vi "solar_log EnQ.vi"(8 "error in (no error)":errorcluster, 9 "Front? (F)":bool, 10 "MSG":string, 11 "Create? (F)":bool) -> (0 "error out":errorcluster, 2 "Created New?":bool, 3 "LogQ":refnum<queue>)   [LabVIEW 2018]
doc: "This obtains and enqueues a message to the logger process. This VI is non-reentrant to avoid multiple opening multiple queue references."
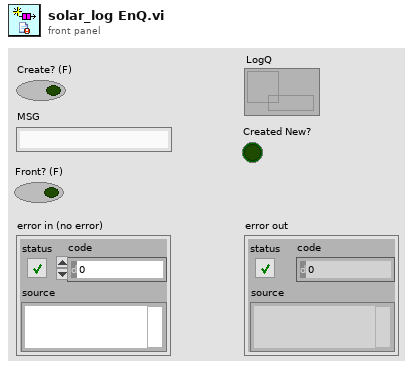
[diagram p1: front panel]
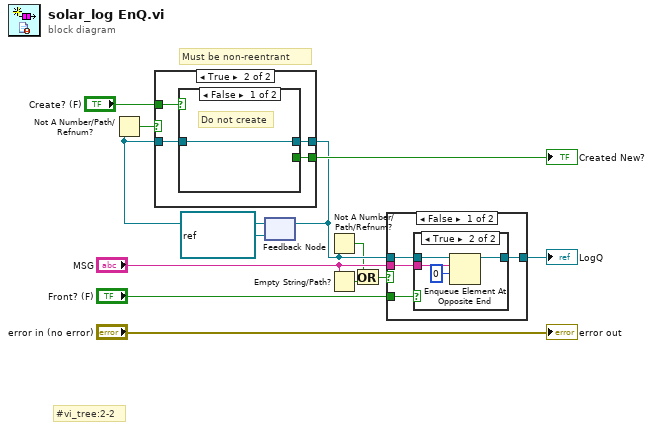
[diagram p0: block diagram]
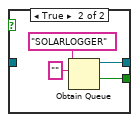
[diagram p3: hidden frame]
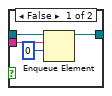
[diagram p4: hidden frame]
diagram:
  # "#vi_tree:2-2"
  # "Must be non-reentrant"
  n1 = feedback #1(refnum<queue> refnum ("queue out")) -> (w12:refnum<queue>)
  n2 = Not A Number/Path/Refnum?(number/path/refnum=w12) -> (NaN/Path/Refnum?=w3:bool)
  n3 = case shown="True" w3 {
    tunnel: [_ w18] -> w13
    tunnel: [w14 w17] -> w9
    tunnel: w12 -> [w14 w15]
    tunnel: "Create? (F)" -> [_ w16]
    frame False {
    }
    frame True {
      n4 = case shown="False" w16 {
        tunnel: [_ w21] -> w18
        tunnel: [w19 w20] -> w17
        tunnel: w15 -> [w19 _]
        frame False {
          # "Do not create"
        }
        frame True {
          n5 = Obtain Queue(name (unnamed)="SOLARLOGGER", element data type="") -> (queue out=w20:refnum<queue>, created new?=w21:bool)  [unwired: 3 in, 1 out]
        }
      }
    }
  }
  "Created New?" <- w13
  n6 = feedback-in #1(w9) -> ()
  n7 = Not A Number/Path/Refnum?(number/path/refnum=w9) -> (NaN/Path/Refnum?=w6:bool)
  n8 = Empty String/Path?(string/path="MSG") -> (empty?=w7:bool)
  n9 = Or(x=w6, y=w7) -> (x .or. y?=w5:bool)
  n10 = case shown="False" w5 {
    tunnel: "MSG" -> [w27 _]
    tunnel: [w26 w36] -> w1
    tunnel: w9 -> [w25 w36]
    tunnel: "Front? (F)" -> [w24 _]
    frame False {
      n11 = case shown="True" w24 {
        tunnel: w27 -> [w30 w33]
        tunnel: [w29 w34] -> w26
        tunnel: w25 -> [w28 w35]
        frame False {
          n12 = Enqueue Element(queue=w28, element=w30, timeout in ms (-1)=0) -> (queue out=w29:refnum<queue>)  [unwired: 1 in, 2 out]
        }
        frame True {
          n13 = Enqueue Element At Opposite End(queue=w35, element=w33, timeout in ms (-1)=0) -> (queue out=w34:refnum<queue>)  [unwired: 1 in, 2 out]
        }
      }
    }
    frame True {
    }
  }
  "LogQ" <- w1
  "error out" <- "error in (no error)"
